vi "Read Multipage ImageJ TIFF Stack.vi"(7 "ImageJ Tif Path":path) -> (4 "U8 Stack":u8[][][](array[numeric]), 8 "U16 Stack":u16[][][](array[numeric]), 13 "Image Info":T1, 15 "U8 Image?":bool)   [LabVIEW 2016]
uses:
  ImageJ TIF Type Defs/TIF Read Image Information.ctl
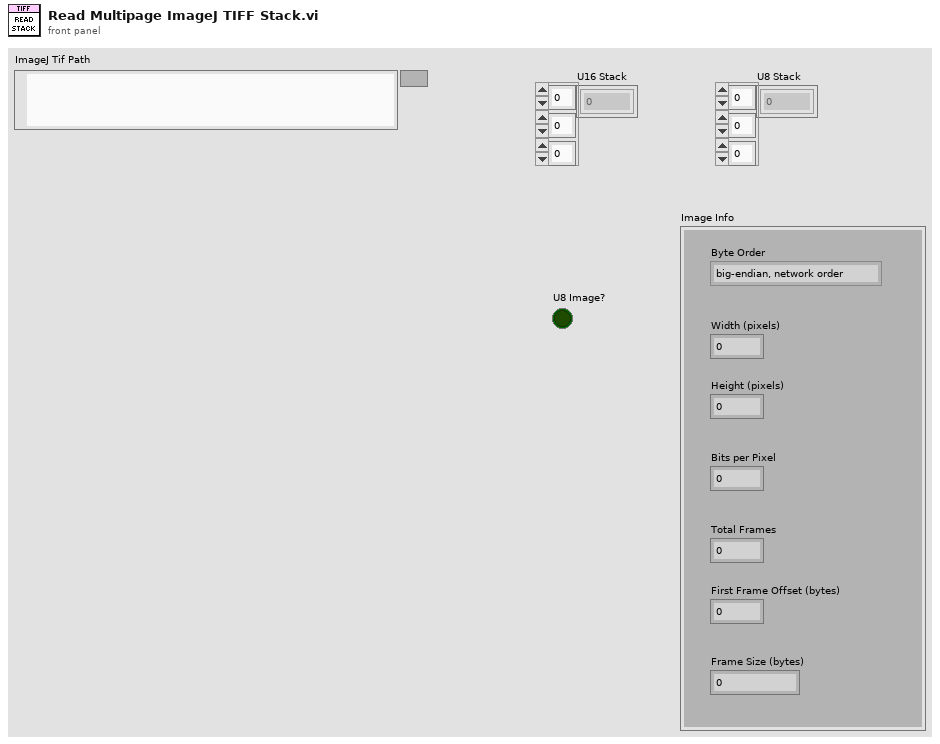
[diagram p1: front panel]
types:
  T1 = typedef "TIF Read Image Information.ctl" = cluster{"Byte Order":enum16{"big-endian, network order", "native, host order", "little-endian"}, "Width (pixels)":i32, "Height (pixels)":i32, "Bits per Pixel":u8, "Total Frames":u32, "First Frame Offset (bytes)":u32, "Frame Size (bytes)":u32}
  T2 = enum16{"big-endian, network order", "native, host order", "little-endian"}
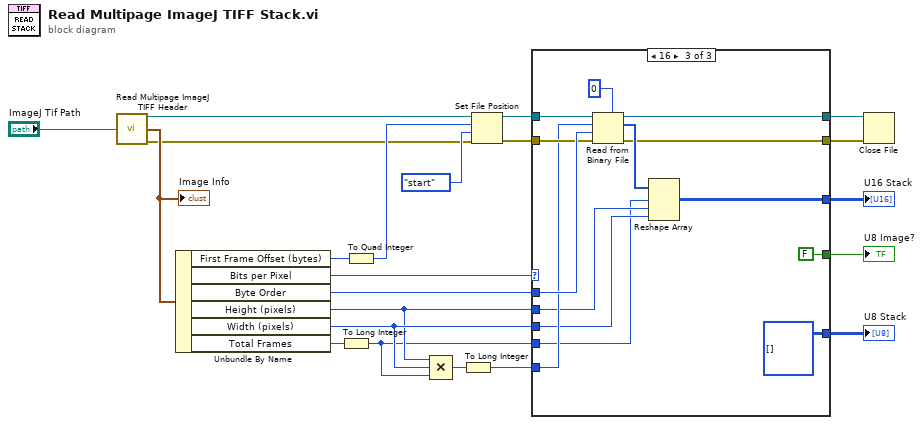
[diagram p0: block diagram]
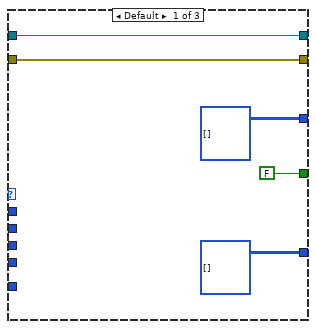
[diagram p2: hidden frame]
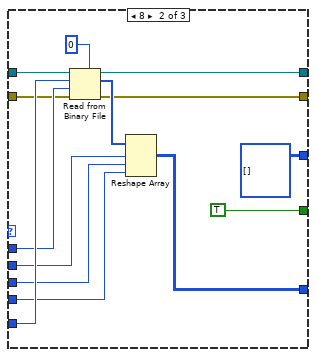
[diagram p3: hidden frame]
diagram:
  n1 = call "Read Multipage ImageJ TIFF Header.vi"("TIFF Path"="ImageJ Tif Path") -> ("TIF Ref"=w20:refnum<file>, "Image Info"=w21:T1, "Error"=w13:errorcluster)  [unwired: 12 in]
  "Image Info" <- w21
  n2 = Unbundle By Name(w21) -> ("First Frame Offset (bytes)"=w18:u32, "Bits per Pixel"=w15:u8, "Byte Order"=w6:T2, "Height (pixels)"=w3:i32, "Width (pixels)"=w4:i32, "Total Frames"=w5:u32)
  n3 = To Long Integer(number=w5) -> (32bit integer=w2:i32)
  n4 = To Quad Integer(1:w18) -> (0:w17:i64)
  n5 = Compound Arithmetic op=MULTIPLY(w3, w4, w2) -> (w1:i32)
  n6 = To Long Integer(number=w1) -> (32bit integer=w12:i32)
  n7 = Set File Position(offset (in bytes) (0)=w17, refnum=w20, from (0:start)=enum16{"start", "end", "current"}."start", error in=w13) -> (refnum out=w16:refnum<file>, error out=w14:errorcluster)
  n8 = case shown="16" w15 {
    tunnel: w16 -> [w27 w41 w55]
    tunnel: w12 -> [_ w39 w45]
    tunnel: w6 -> [_ w38 w53]
    tunnel: w14 -> [w26 w37 w52]
    tunnel: w3 -> [_ w35 w43]
    tunnel: w4 -> [_ w34 w44]
    tunnel: [w27 w33 w50] -> w11
    tunnel: [w26 w32 w49] -> w10
    tunnel: [FALSE TRUE FALSE] -> w9
    tunnel: w2 -> [_ w30 w42]
    tunnel: [u16[][][] [] u16[][][] [] w47] -> w8
    tunnel: [u8[][][] [] w29 u8[][][] []] -> w7
    frame Default {
    }
    frame 8 {
      n9 = Read from Binary File(5:u8 0, 8:w37, 9:w38, 10:w39, 11:w41) -> (0:w32:errorcluster, 2:w36:u8[], 3:w33:refnum<file>)  [unwired: 1 in, 1 out]
      n10 = Reshape Array(w36, w35, w34, w30) -> (w29:u8[][][])
    }
    frame 16 {
      n11 = Read from Binary File(5:u16 0, 8:w52, 9:w53, 10:w45, 11:w55) -> (0:w49:errorcluster, 2:w51:u16[], 3:w50:refnum<file>)  [unwired: 1 in, 1 out]
      n12 = Reshape Array(w51, w42, w43, w44) -> (w47:u16[][][])
    }
  }
  "U8 Image?" <- w9
  "U16 Stack" <- w8
  "U8 Stack" <- w7
  n13 = Close File(refnum=w11, error in=w10) -> ()  [unwired: 2 out]
